vi "speech.vi"() -> ()   [LabVIEW 2020]
uses:
  System.Speech
panel:
  in  "String":string
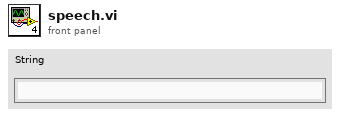
[diagram p1: front panel]
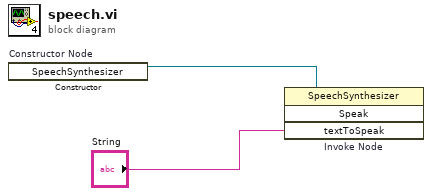
[diagram p0: block diagram]
diagram:
  n1 = constructor on="Constructor Node" class="SpeechSynthesizer"() -> (reference out=w2:refnum<k24>)  [unwired: 3 in, 2 out]
  n2 = invoke on="Invoke Node" class="SpeechSynthesizer" method="Speak"(reference=w2, "textToSpeak"="String") -> ()  [unwired: 2 in, 4 out]
